vi "Komponentenauswahl aus SPAN Idx.vi"(8 "Fehler (Eingang, kein Fehler)":errorcluster, 11 "Span Iindex":i32) -> (0 "Fehler (Ausgang)":errorcluster, 3 "Komponentenauswahl":T1(array[cluster]))   [LabVIEW 2020, in "Linearisierung v2.lvlib" / "SpanEinstellungen.lvlib"]
uses:
  SpanEinstellungen.lvlib
  Aktion FGV SpanEinstellungen.ctl
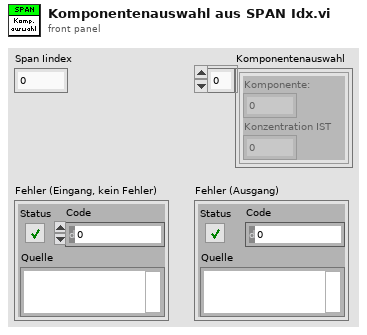
[diagram p1: front panel]
types:
  T1 = cluster{"Komponente:":u16, "Konzentration IST":dbl}[]
  T2 = typedef "Linearisierung v2.lvlib/SpanEinstellungen.lvlib/Aktion FGV SpanEinstellungen.ctl" = enum16{"lesen", "schreiben", "laden", "speichern", "RegisterRef", "automatisch", "init", "PDF Params", "Punkte umkehren"}
  T3 = typedef "Linearisierung v2.lvlib/SpanEinstellungen.lvlib/SpanInletCluster.ctl" = cluster{"Span Inlet Active":T4, "Analysator":T5, "Konfig Gasflasche":T4, "Gasflasche":T6, "Gasflaschen Nr.:":string, "Ablaufdatum":timestamp, "Komponenten":T7, "Zeitdauer Stufen":sgl, "Max Fehler":sgl, "Anzahl Stufen":sgl, "Trägergas":T11, "zusätzliche Zeitdauer Erster Punkt":sgl}
  T4 = typedef "System Einstellungen V2.lvlib/Konfig Gasflasche.ctl" = bool
  T5 = typedef "System Einstellungen V2.lvlib/Analysatoren.ctl" = string
  T6 = typedef "System Einstellungen V2.lvlib/Gasflasche Auswahl.ctl" = u16
  T7 = typedef "Linearisierung v2.lvlib/SpanEinstellungen.lvlib/Komponentencluster mit Formel.ctl" = cluster{"Komponente 1":T8, "Komponente 2":T8, "Komponente 3":T8, "Komponente 4":T8, "Komponente 5":T8}
  T8 = typedef "Linearisierung v2.lvlib/SpanEinstellungen.lvlib/Komponentenauswahl mit Formel.ctl" = cluster{"Komponente:":u16, "Summenformel":T9, "Konzentration IST":dbl, "Einheit":T10, "Genauigkeit":dbl}
  T9 = typedef "String - Eingabefeld.ctl" = string
  T10 = typedef "Linearisierung v2.lvlib/SpanEinstellungen.lvlib/Einheit.ctl" = enum16{"ppm", "%"}
  T11 = typedef "System Einstellungen V2.lvlib/Traegergas.ctl" = string
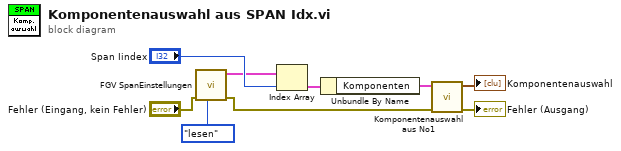
[diagram p0: block diagram]
diagram:
  n1 = call "FGV SpanEinstellungen.vi"("Aktion"=Aktion_FGV_SpanEinstellungen."lesen", "error in (no error)"="Fehler (Eingang, kein Fehler)") -> ("error out"=w2:errorcluster, "SpanInletClusterArray out"=w5:T3[])  [unwired: 5 in, 3 out]
  n2 = Index Array(array=w5, index="Span Iindex") -> (element=w6:T3)
  n3 = Unbundle By Name(w6) -> ("Komponenten"=w7:T7)
  n4 = call "Komponentenauswahl aus No1.vi"("Fehler (Eingang, kein Fehler)"=w2, "Komponente 1"=w7) -> ("Fehler (Ausgang)"=→"Fehler (Ausgang)":errorcluster, "Komponentenauswahl"=→"Komponentenauswahl":T1)  [unwired: 7 in, 1 out]
